vi "StartProcess.vi"(0 "reference in":refnum<class "HPPC.lvclass">, 3 "ms timeout (-1)":i32=-1, 5 "Error In":errorcluster) -> (14 "reference out":refnum<class "HPPC.lvclass">, 15 "EventFromProcess":refnum<user-event>, 16 "timed out":bool, 17 "ProcessViRef":refnum<vi>, 19 "Error Out":errorcluster)   [LabVIEW 2023, in "HPPC.lvclass"]
doc: "Looks up an existing object matching object name or creates a new object and returns a refnum you can use when calling other class methods.\n\nObjects created with this VI should be destroyed using this class Delete VI."
uses:
  HPPC.lvclass
  HPPC.lvclass/HPPC.ctl
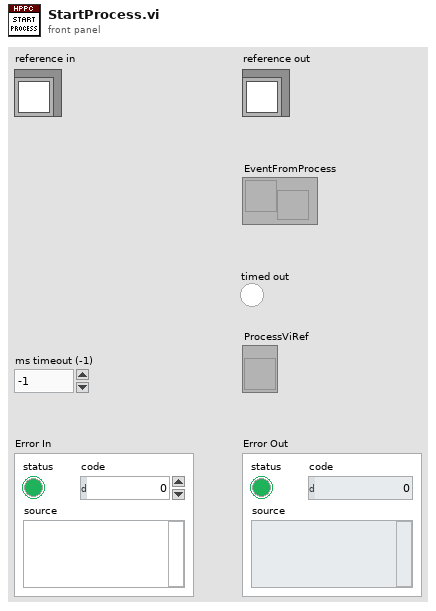
[diagram p1: front panel]
types:
  T1 = enum16{"ReadRepository", "CreateNew", "CreateOrLookUpExisting", "ReadRepositoryAndDestroy"}
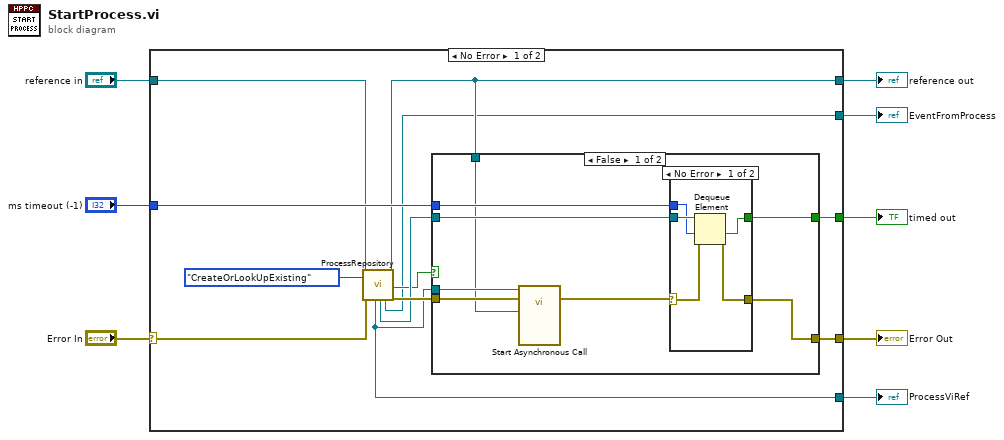
[diagram p0: block diagram]
diagram:
  n1 = case shown="No Error" "Error In" {
    selector: "Error In" -> [w17 w36]
    tunnel: [w18 w36] -> w7
    tunnel: [w14 w37] -> w5
    tunnel: "reference in" -> [w12 w37]
    tunnel: "ms timeout (-1)" -> [w20 _]
    tunnel: [w19 _] -> w3
    tunnel: [w11 _] -> w2
    tunnel: [w9 _] -> w1
    frame No Error {
      n2 = call "ProcessRepository.vi"("reference in"=w12, "Action(ReadRepository)"=T1."CreateOrLookUpExisting", "Error In"=w17) -> ("ProcessViRef"=w9:refnum<vi>, "ProcessSyncQueue"=w15:refnum<queue>, "EventFromProcess"=w11:refnum<user-event>, "reference out"=w14:refnum<class "HPPC.lvclass">, "ProcessAlreadyStarted"=w13:bool, "Error Out"=w16:errorcluster)  [unwired: 9 in, 2 out]
      n3 = case shown="False" w13 {
        tunnel: w20 -> [w28 _]
        tunnel: [w27 _] -> w19
        tunnel: [w26 w35] -> w18
        tunnel: w16 -> [w24 w35]
        tunnel: w9 -> [w23 _]
        tunnel: w15 -> [w25 _]
        tunnel: w14 -> [w22 _]
        frame False {
          n4 = call-by-ref "Start Asynchronous Call"(reference=w23, error in=w24, "reference in"=w22) -> (error out=w21:errorcluster)  [unwired: 17 in, 3 out]
          n5 = case shown="No Error" w21 {
            tunnel: w25 -> [w33 _]
            tunnel: w28 -> [w31 _]
            tunnel: [w32 _] -> w27
            selector: w21 -> [w30 w34]
            tunnel: [w29 w34] -> w26
            frame No Error {
              n6 = Dequeue Element(queue=w33, timeout in ms (-1)=w31, error in (no error)=w30) -> (timed out?=w32:bool, error out=w29:errorcluster)  [unwired: 2 out]
            }
            frame Error {
            }
          }
        }
        frame True {
          # "Process Already started.\nThis option will only be used togeather with the\naction: \"CreateOrLookUpExisting\""
        }
      }
    }
    frame Error {
    }
  }
  "Error Out" <- w7
  "reference out" <- w5
  "timed out" <- w3
  "EventFromProcess" <- w2
  "ProcessViRef" <- w1
